vi "Read Binary Address.vi"(8 "error in (no error)":errorcluster, 11 "Addressing Mode in":refnum<class "Addressing Mode.lvclass">) -> (0 "error out":errorcluster, 2 "Binary Address":i16[](array[numeric]), 3 "Addressing Mode out":refnum<class "Addressing Mode.lvclass">)   [LabVIEW 2020, in "Addressing Mode.lvclass"]
uses:
  Addressing Mode.lvclass
  Addressing Mode.lvclass/Addressing Mode.ctl
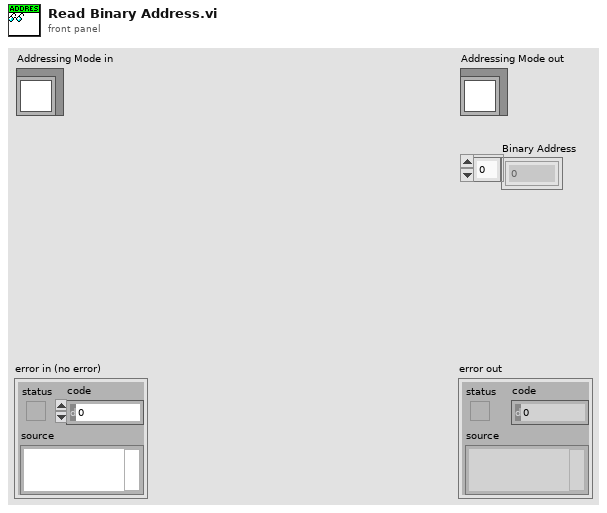
[diagram p1: front panel]
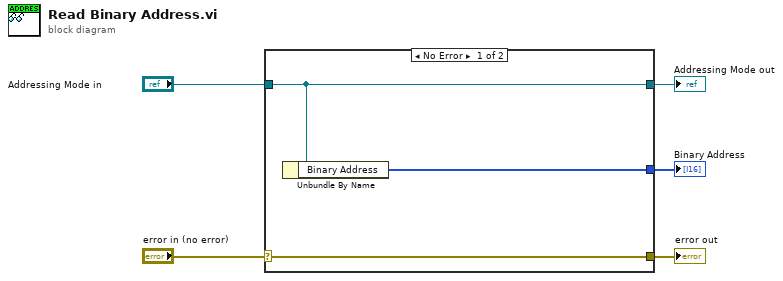
[diagram p0: block diagram]
diagram:
  n1 = case shown="No Error" "error in (no error)" {
    selector: "error in (no error)" -> [w8 w9]
    tunnel: [w8 w9] -> w4
    tunnel: [w7 w10] -> w2
    tunnel: "Addressing Mode in" -> [w7 w10]
    tunnel: [w6 _] -> w1
    frame No Error {
      n2 = Unbundle By Name(w7) -> ("Binary Address"=w6:i16[])
    }
    frame Error {
    }
  }
  "error out" <- w4
  "Addressing Mode out" <- w2
  "Binary Address" <- w1
